vi "Get Buffer Info.vi"(8 "error in (no error)":errorcluster, 11 "Buffer-Mapped in":refnum<class "Buffer-Mapped.lvclass">) -> (0 "error out":errorcluster, 1 "Byte Stream (Do Not Delete)":refnum<data-value>, 2 "Y Resolution":i32, 3 "X Resolution":i32, 4 "Image Info.Bytes to Copy":u64)   [LabVIEW 2020, in "Buffer-Mapped.lvclass"]
uses:
  Buffer-Mapped.lvclass
  Buffer-Mapped.lvclass/Buffer-Mapped.ctl
  Buffer/Buffer.lvclass
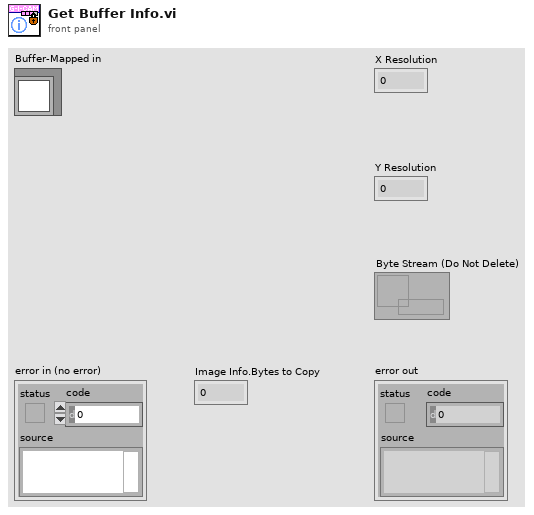
[diagram p1: front panel]
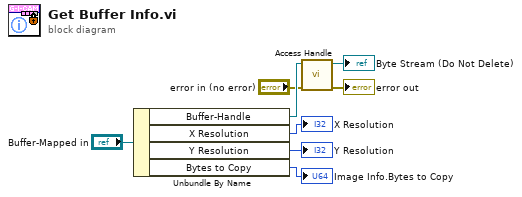
[diagram p0: block diagram]
diagram:
  n1 = Unbundle By Name("Buffer-Mapped in") -> ("Buffer-Handle"=w4:refnum<class "Buffer.lvclass">, "X Resolution"=→"X Resolution":i32, "Y Resolution"=→"Y Resolution":i32, "Bytes to Copy"=→"Image Info.Bytes to Copy":u64)
  n2 = call "Access Handle.vi"("error in (no error)"="error in (no error)", "Buffer"=w4) -> ("error out"=→"error out":errorcluster, "Handle"=→"Byte Stream (Do Not Delete)":refnum<data-value>)  [unwired: 8 in]
